vi "Intake Arm Controller.vi"(8 "error in":errorcluster) -> ()   [LabVIEW 2020]
doc: "This VI executes continuously carrying out the current operation and responding to updates or new operations. It will often contain the timing or control code that is difficult to place directly in TeleOp. This VI generally opens all sensors and motors and isolates the rest of the robot code from knowing how the operations are carried out."
uses:
  <vilib>/Rock Robotics/WPI/Framework/Completion Status.ctl
  Intake Arm Setpoints.ctl
  Intake Arm Operations.ctl
  <vilib>/Rock Robotics/WPI/SafetyOutput/WPI_SafetyOutputConfigMenu.ctl
  <vilib>/Rock Robotics/WPI/Solenoid/WPI_SolenoidSetEnum.vi
panel:
  in  "Interactive Values":T1
  out "Current\nCmd":string
  in  "Buttons":cluster{"Execute Cmd":bool, "Abort Cmd":bool}
  out "Command Timing":cluster{"Start Time (ms)":u32, "Iterations":i32}
  out "Status":T3
  # "Tip: It may be helpful to observe inputs and sensor values.\nYou may also want to display tuning or debugging controls."
  # "Interactive Command: You may fill in the settings for a command\nand schedule it with the Execute button. You can observe and abort\nany command while fine tuning the code for the controller."
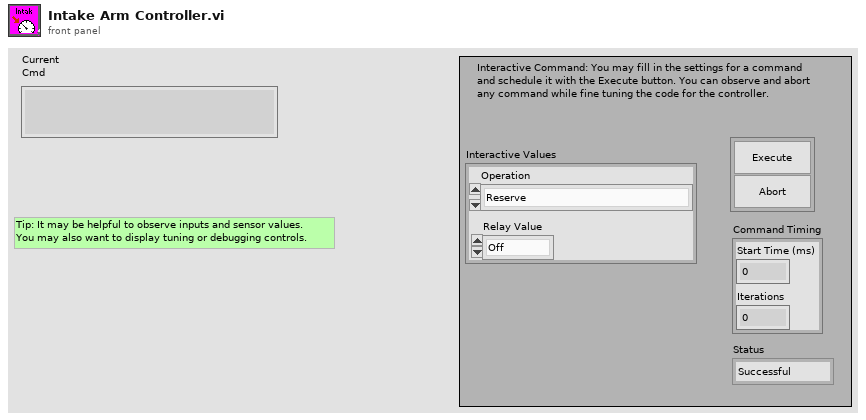
[diagram p1: front panel]
types:
  T1 = typedef "Intake Arm Setpoints.ctl" = cluster{"Operation":T2, "Relay Value":enum16{"Off", "On", "Forward", "Reverse"}}
  T2 = typedef "Intake Arm Operations.ctl" = enum16{"Reserve", "Read Current", "Immediate", "Intake Arm Immediate"}
  T3 = typedef "Completion Status.ctl" = enum16{"Successful", "Aborted", "Incomplete"}
  T4 = typedef "WPI_SafetyOutputConfigMenu.ctl" = enum16{"Enable", "Disable"}
  T5 = typedef "WPI_SolenoidDevRef.ctl" = cluster{"DevStatus":errorcluster, "Pneumatics Control Module":u8, "Forward Solenoid Channel":T6, "Reverse Solenoid Channel":T6}
  T6 = typedef "WPI_SolenoidChannel.ctl" = enum8{"Solenoid 0", "Solenoid 1", "Solenoid 2", "Solenoid 3", "Solenoid 4", "Solenoid 5", "Solenoid 6", "Solenoid 7", "Solenoid 8", "Solenoid 9", "Solenoid 10", "Solenoid 11", "Solenoid 12", "Solenoid 13", "Solenoid 14", "Solenoid 15", "Invalid"}
  T7 = typedef "Command Status Info.ctl" = cluster{"Name":string, "Status":T3, "notifier out":T8}
  T8 = typedef "Completion Notifier.ctl" = refnum<notifier>
  T9 = cluster{"Current Command":T1, "Command Timing":cluster{"Start Time (ms)":u32, "Iterations":i32}, "Command Arguments":cluster{"Command Info":T7, "Description":string, "Default Command":T1, "queue out":refnum<queue>, "Subsystem Name":string}}
  T10 = cluster{u32, "Relay Value":enum16{"Off", "On", "Forward", "Reverse"}}
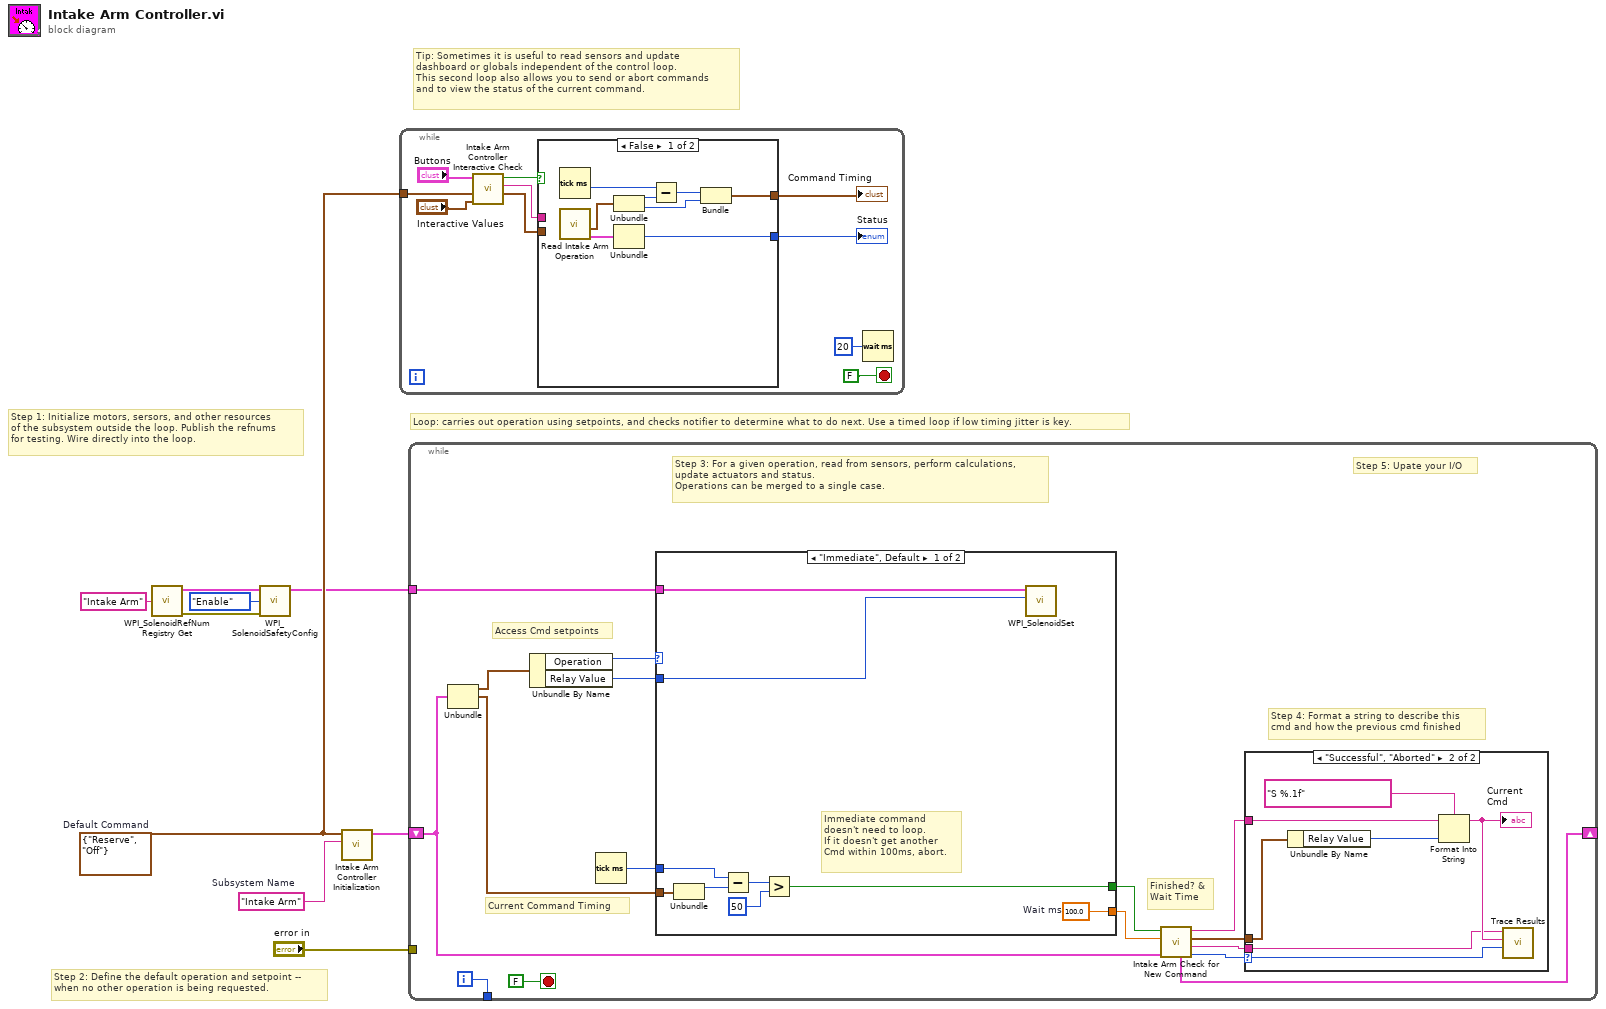
[diagram p0: block diagram]
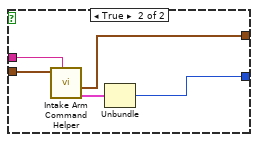
[diagram p2: hidden frame]
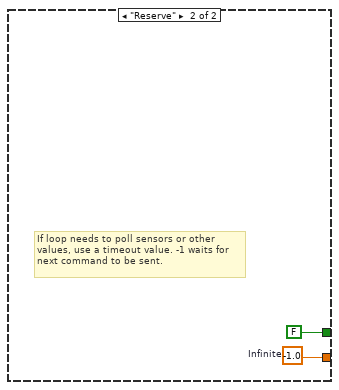
[diagram p4: hidden frame]
diagram:
  w6 = T1 {"Operation"=enum."Reserve", "Relay Value"=enum."Off"}  # Default Command
  w7 = "Intake Arm"  # Subsystem Name
  # "Tip: Sometimes it is useful to read sensors and update\ndashboard or globals independent of the control loop.\nThis second loop also allows you to send or abort commands\nand to view the status of the current command."
  # "Step 2: Define the default operation and setpoint --\nwhen no other operation is being requested."
  # "Step 1: Initialize motors, sersors, and other resources\nof the subsystem outside the loop. Publish the refnums\nfor testing. Wire directly into the loop."
  # "Loop: carries out operation using setpoints, and checks notifier to determine what to do next. Use a timed loop if low timing jitter is key."
  n1 = call <vilib>:"WPI_SolenoidRefNum Registry Get.vi"("refnum name"="Intake Arm") -> ("error out"=w4:errorcluster, "SolenoidDevRef"=w5:T5)  [unwired: 9 in]
  n2 = call <vilib>:"WPI_SolenoidSafetyConfig.vi"("error in (no error)"=w4, "mode"=WPI_SafetyOutputConfigMenu."Enable", "SolenoidDevRef"=w5) -> ("SolenoidDevRef"=w1:T5)  [unwired: 7 in, 1 out]
  n3 = call "Intake Arm Controller Initialization.vi"("Subsystem Name"=w7, "Default Command"=w6) -> ("Current Command"=w8:T9)  [unwired: 9 in]
  n4 = while {
    tunnel: w6 -> [w16]
    stop <- FALSE stop-if-true
    n5 = call "Intake Arm Controller Interactive Check.vi"("Interactive Command in"="Interactive Values", "Default Command"=w16, "Buttons"="Buttons") -> ("Interactive Command out"=w13:T1, "Trace String"=w14:string, "Schedule"=w15:bool)  [unwired: 6 in]
    n6 = case shown="False" w15 {
      tunnel: [w27 w32] -> w12
      tunnel: w13 -> [_ w30]
      tunnel: [w23 w28] -> w11
      tunnel: w14 -> [_ w31]
      frame False {
        n7 = Tick Count (ms)() -> (millisecond timer value=w22:u32)
        n8 = call "Read Intake Arm Operation.vi"() -> ("Command Info"=w20:T7, "SubSystem Data"=w21:T1)  [unwired: 9 in, 1 out]
        n9 = Unbundle(w21) -> ("Operation"=w26:T2, "Relay Value"=w24:enum16{"Off", "On", "Forward", "Reverse"})
        n10 = Unbundle(w20) -> ("Status"=w27:T3)  [unwired: 2 out]
        n11 = Subtract(x=w22, y=w26) -> (x-y=w25:u32)
        n12 = Bundle(w25, "Relay Value"=w24) -> (w23:T10)  [unwired: 1 in]
      }
      frame True {
        n13 = call "Intake Arm Command Helper.vi"("Description"=w31, "SubSystem Data"=w30) -> ("Command Info Out"=w29:T7, "Command Timing"=w28:cluster{"Start Time (ms)":u32, "Iterations":i32})  [unwired: 7 in, 1 out]
        n14 = Unbundle(w29) -> ("Status"=w32:T3)  [unwired: 2 out]
      }
    }
    "Status" <- w12
    "Command Timing" <- w11
    n15 = Wait (ms)(milliseconds to wait=u32 20) -> ()  [unwired: 1 out]
  }
  n16 = while {
    shift-right: [w41] -> _
    shift-left: w8 -> [w34]
    tunnel: [w47] -> _
    tunnel: "error in" -> [_]
    tunnel: w1 -> [w33]
    i -> [w47]
    stop <- FALSE stop-if-true
    # "Step 5: Upate your I/O"
    # "Step 4: Format a string to describe this\ncmd and how the previous cmd finished"
    # "Current Command Timing"
    # "Access Cmd setpoints"
    # "Finished? &\nWait Time"
    # "Step 3: For a given operation, read from sensors, perform calculations,\nupdate actuators and status.\nOperations can be merged to a single case."
    n17 = Unbundle(w34) -> ("Current Command"=w46:T1, "Command Timing"=w42:cluster{"Start Time (ms)":u32, "Iterations":i32})  [unwired: 1 out]
    n18 = Unbundle By Name(w46) -> ("Operation"=w45:T2, "Relay Value"=w44:enum16{"Off", "On", "Forward", "Reverse"})
    n19 = Tick Count (ms)() -> (millisecond timer value=w43:u32)
    n20 = case shown="\"Immediate\", Default" w45 {
      tunnel: [w64 w66] -> w39
      tunnel: [w58 FALSE ("ignore previous (F)")] -> w40
      tunnel: w42 -> [w60 _]
      tunnel: w44 -> [w56 _]
      tunnel: w43 -> [w59 _]
      tunnel: w33 -> [w57 _]
      frame "Immediate", Default {
        w64 = 100.0  # Wait ms
        # "Immediate command\ndoesn't need to loop.\nIf it doesn't get another\nCmd within 100ms, abort."
        n21 = Unbundle(w60) -> ("Start Time (ms)"=w63:u32)  [unwired: 1 out]
        n22 = Subtract(x=w59, y=w63) -> (x-y=w62:u32)
        n23 = Greater?(x=w62, y=u8 50 ("Left Motor")) -> (0:w58:bool)
        n24 = call-poly <vilib>:"WPI_SolenoidSet.vi"("Value"=w56, "SolenoidDevRef"=w57) -> ()  [unwired: 8 in, 2 out]
      }
      frame "Reserve" {
        w66 = -1.0  # Infinite
        # "If loop needs to poll sensors or other\nvalues, use a timeout value. -1 waits for\nnext command to be sent."
      }
    }
    n25 = call "Intake Arm Check for New Command.vi"("Current Command"=w34, "Wait time (ms)"=w39, "Finished?"=w40) -> ("Completion"=w35:T3, "Subsystem Name"=w36:string, "Current Command"=w37:T1, "Initial Trace String"=w38:string, "NextCommand"=w41:T9)  [unwired: 4 in]
    n26 = case shown="\"Successful\", \"Aborted\"" w35 {
      selector: w35 -> [_ w55]
      tunnel: w38 -> [_ w51]
      tunnel: w37 -> [_ w52]
      tunnel: w36 -> [_ w49]
      frame "Incomplete", Default {
        # "Continuing current command"
      }
      frame "Successful", "Aborted" {
        # "Report and setup for next command"
        n27 = Unbundle By Name(w52) -> ("Relay Value"=w54:enum16{"Off", "On", "Forward", "Reverse"})
        n28 = Format Into String(format string="S %.1f", initial string=w51, w54) -> (resulting string=w50:string)  [unwired: 1 in, 1 out]
        "Current\nCmd" <- w50
        n29 = call <vilib>:"Trace Results.vi"("Status of previous command"=w55, "Description"=w50, "Subsystem"=w49) -> ()  [unwired: 9 in]
      }
    }
  }
